vi "DAQ_PIC.vi"() -> ()   [LabVIEW 2016]
panel:
  out "subarray":bool[](array[boolean])
  in  "Stop Button":bool
  in  "Array":bool[](array[boolean])
  out "Cierre":bool
  out "PIPE_OUT":i32
  out "PIPE_IN":i32
  out "PIPES":cluster{"PIPE_IN":i32, "PIPE_OUT":i32}
  out "NDISPOSITIVOS":i32
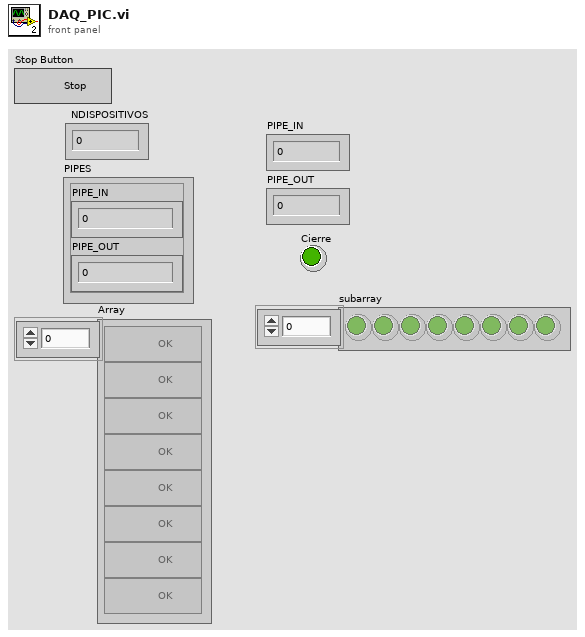
[diagram p1: front panel]
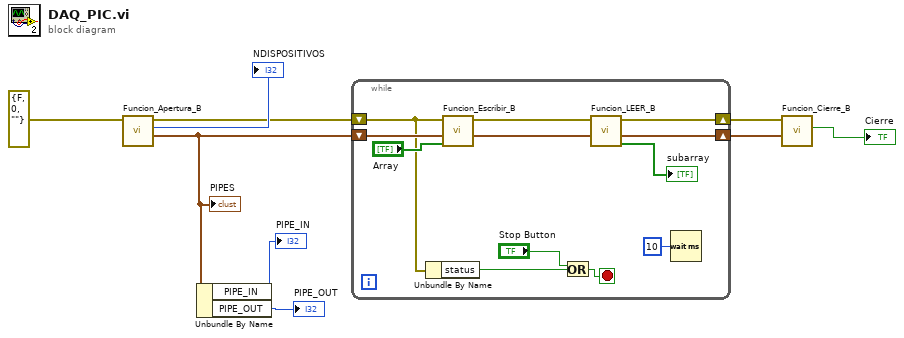
[diagram p0: block diagram]
diagram:
  n1 = call "Funcion_Apertura_B.vi"("error in (no error)"=errorcluster {"status"=FALSE, "code"=0, "source"=""}) -> ("PIPES"=w3:cluster{"PIPE_IN":i32, "PIPE_OUT":i32}, "NDISPOSITIVOS"=→"NDISPOSITIVOS":i32, "error out"=w4:errorcluster)  [unwired: 8 in]
  "PIPES" <- w3
  n2 = Unbundle By Name(w3) -> ("PIPE_IN"=→"PIPE_IN":i32, "PIPE_OUT"=→"PIPE_OUT":i32)
  n3 = while {
    shift-right: [w12] -> w2
    shift-left: w4 -> [w17]
    shift-right: [w13] -> w1
    shift-left: w3 -> [w20]
    stop <- w18 stop-if-true
    n4 = Unbundle By Name(w17) -> ("status"=w16:bool)
    n5 = call "Funcion_Escribir_B.vi"("Array"="Array", "PIPES ENTRADA"=w20, "error in (no error)"=w17) -> ("PIPES SALIDA"=w14:cluster{"PIPE_IN":i32, "PIPE_OUT":i32}, "error out"=w15:errorcluster)  [unwired: 7 in]
    n6 = Or(x="Stop Button", y=w16) -> (x .or. y?=w18:bool)
    n7 = call "Funcion_LEER_B.vi"("PIPES ENTRADA"=w14, "error in (no error)"=w15) -> ("subarray"=→"subarray":bool[], "PIPES SALIDA"=w13:cluster{"PIPE_IN":i32, "PIPE_OUT":i32}, "error out"=w12:errorcluster)  [unwired: 7 in]
    n8 = Wait (ms)(milliseconds to wait=u32 10) -> ()  [unwired: 1 out]
  }
  n9 = call "Funcion_Cierre_B.vi"("PIPES"=w1, "error in (no error)"=w2) -> ("Cierre"=→"Cierre":bool)  [unwired: 8 in, 1 out]
